vi "When Read.vi"(0 "error out":errorcluster, 2 "Data Out":u8[](array[numeric]) format="%.0x", 11 "I2C Bus in":refnum<class "Mock I2C Bus.lvclass">) -> (3 "I2C Bus out":refnum<class "Mock I2C Bus.lvclass">)   [LabVIEW 2020, in "Mock I2C Bus.lvclass"]
uses:
  Mock I2C Bus.lvclass
  C:/Program Files (x86)/National Instruments/LabVIEW 2020/vi.lib/Astemes/LMock/Mock.lvclass
  <vilib>/Astemes/LMock/Mock.lvclass
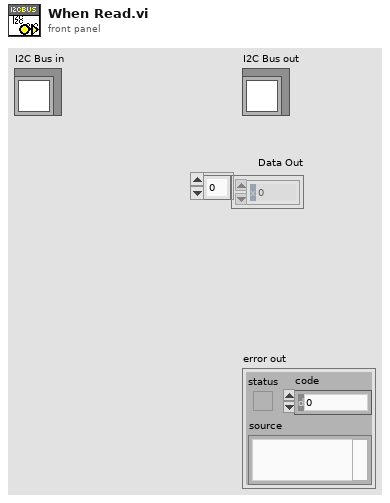
[diagram p1: front panel]
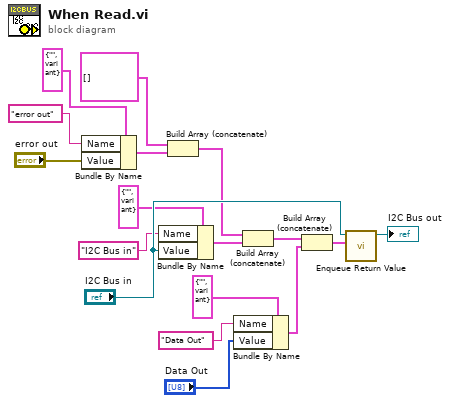
[diagram p0: block diagram]
diagram:
  n1 = Bundle By Name(cluster=cluster{"Name":string, "Value":variant} {"Name"="", "Value"=variant} ("element"), "Name"="error out", "Value"="error out") -> (w5:cluster{"Name":string, "Value":variant})
  n2 = Bundle By Name(cluster=cluster{"Name":string, "Value":variant} {"Name"="", "Value"=variant} ("element"), "Name"="I2C Bus in", "Value"="I2C Bus in") -> (w3:cluster{"Name":string, "Value":variant})
  n3 = Build Array (concatenate)(cluster{"Name":string, "Value":variant}[] [] ("Control Values"), w5) -> (w10:cluster{"Name":string, "Value":variant}[])
  n4 = Bundle By Name(cluster=cluster{"Name":string, "Value":variant} {"Name"="", "Value"=variant} ("element"), "Name"="Data Out", "Value"="Data Out") -> (w1:cluster{"Name":string, "Value":variant})
  n5 = Build Array (concatenate)(w10, w3) -> (w12:cluster{"Name":string, "Value":variant}[])
  n6 = Build Array (concatenate)(w12, w1) -> (w15:cluster{"Name":string, "Value":variant}[])
  n7 = call <vilib>:"Enqueue Return Value.vi"("Indicator Values"=w15, "Mock In"="I2C Bus in") -> ("Mock Out"=→"I2C Bus out":refnum<class "Mock I2C Bus.lvclass">)  [unwired: 8 in, 1 out]
